vi "Open nested object parameters.vi"(8 "error in (no error)":errorcluster, 10 "Object name":string, 11 "Mag Lab Measure Base in":refnum<class "Mag Lab Measure Base.lvclass">) -> (0 "error out":errorcluster, 3 "Mag Lab Measure Base out":refnum<class "Mag Lab Measure Base.lvclass">)   [LabVIEW 2015, in "Mag Lab Measure Base.lvclass"]
uses:
  Mag Lab Measure Base.lvclass
  Mag Lab Measure Base.lvclass/Mag Lab Measure Base.ctl
  <vilib>/ActorFramework/Actor/Actor.lvclass/Actor.ctl
  Mag Lab Measure Base Messages/Open sub-object parameters Msg/Open nested object parameters Msg.lvclass/Open nested object parameters Msg.ctl
  <vilib>/ActorFramework/Message Enqueuer/Message Enqueuer.lvclass/Message Enqueuer.ctl
  <vilib>/ActorFramework/Message Enqueuer/Enqueue.vi
  <vilib>/ActorFramework/Message Priority Queue/Priority Enqueue.vi
  Mag Lab Measure Base Messages/Open sub-object parameters Msg/Open nested object parameters Msg.lvclass
  Mag Lab Root Messages/Open Front Panel Msg/Open Front Panel Msg.lvclass
  Mag Lab Error Handler/Mag Lab Error Handler.lvclass
  <vilib>/ActorFramework/Actor/Actor.lvclass
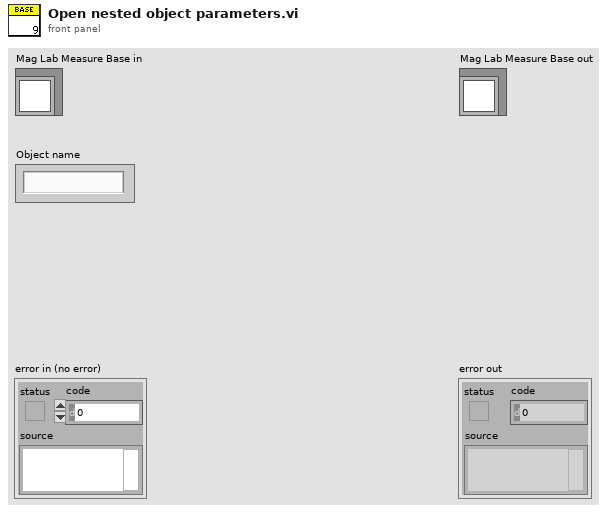
[diagram p1: front panel]
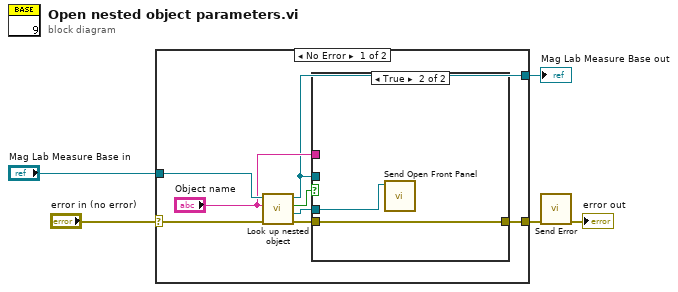
[diagram p0: block diagram]
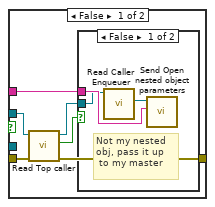
[diagram p2: hidden frame]
diagram:
  n1 = case shown="No Error" "error in (no error)" {
    selector: "error in (no error)" -> [w12 w26]
    tunnel: [w6 w26] -> w2
    tunnel: [w8 w25] -> w3
    tunnel: "Mag Lab Measure Base in" -> [w13 w25]
    frame No Error {
      n2 = call "Look up nested object.vi"("error in (no error)"=w12, "Object name"="Object name", "Mag Lab Measure Base in"=w13) -> ("error out"=w7:errorcluster, "Object Queue"=w10:refnum<class "Message Enqueuer.lvclass">, "Found?"=w11:bool, "Mag Lab Measure Base out"=w8:refnum<class "Mag Lab Measure Base.lvclass">)  [unwired: 5 in]
      n3 = case shown="True" w11 {
        tunnel: w10 -> [_ w23]
        tunnel: w8 -> [w18 _]
        tunnel: "Object name" -> [w19 _]
        tunnel: w7 -> [w15 w24]
        tunnel: [w14 w24] -> w6
        frame False {
          n4 = call "Read Top caller.vi"("error in (no error)"=w15, "Mag Lab Measure Base in"=w18) -> ("error out"=w14:errorcluster, "Top caller"=w16:bool, "Mag Lab Measure Base out"=w17:refnum<class "Mag Lab Measure Base.lvclass">)  [unwired: 7 in]
          n5 = case shown="False" w16 {
            tunnel: w19 -> [w22 _]
            tunnel: w17 -> [w20 _]
            frame False {
              # "Not my nested \nobj, pass it up\n to my master"
              n6 = call <vilib>:"Read Caller Enqueuer.vi"("Actor"=w20) -> ("Caller Enqueuer"=w21:refnum<class "Message Enqueuer.lvclass">)  [unwired: 10 in]
              n7 = call "Send Open nested object parameters.vi"("Object name"=w22, "Message Enqueuer"=w21) -> ()  [unwired: 8 in, 2 out]
            }
            frame True {
            }
          }
        }
        frame True {
          n8 = call "Send Open Front Panel.vi"("Message Enqueuer"=w23) -> ()  [unwired: 9 in, 2 out]
        }
      }
    }
    frame Error {
    }
  }
  "Mag Lab Measure Base out" <- w3
  n9 = call "Send Error.vi"("error in (no error)"=w2) -> ("error out"=→"error out":errorcluster)  [unwired: 9 in, 1 out]
